vi "SPI_1203v7.vi"() -> ()   [LabVIEW 2018]
uses:
  <vilib>/ni845x/ni845x.llb/ni845xControl.ctl
  <vilib>/ni845x/ni845x.llb/ni845xSpiStreamConfiguration.ctl
  <vilib>/ni845x/ni845x.llb/NI-845x SPI Script Us Delay.vi
  <vilib>/ni845x/ni845x.llb/NI-845x Close Device Reference.vi
  <resource>/objmgr/NI845x.rc
  <vilib>/ptbypt/NI_PtbyPt.lvlib
panel:
  out "СКО":dbl
  out "СЗС":dbl
  in  "Расчет":bool
  in  "ПРИМЕЧАНИЕ":string="1"
  in  "Сохранить кадр":bool
  in  "Frames":path=path "C:/LabView_PRJ/23011_UIC1203R/LabView_PRJ/Frames"
  in  "Waveform1:Timing:T4(drdyA->csA)":u32=20
  in  "RST":bool
  out "Numeric":u32=1
  out "RX BUFFER":string="B0\t58\t75\t52\t00\t00\t00\t00\tB0\t58\t79\t54\t00\t00\t00\t00\tB0\t58\t7D\t55\t00\t00\t00\t00\tB0\t58\t81\t52\t00\t00\t00\t00\tB0\t58\t85\t52\t00\t00\t00\t00\tB0\t58\t89\t50\t00\t00\t00\t00\tB0\t58\t8D\t53\t00\t00\t00\t00\tB0\t58\t91\t4B\t00\t00\t00\t00\tB0\t58\t95\t54\t00\t00\t00\t00\tB0\t58\t99\t4F\t00\t00\t00\t00\tB0\t58\t9D\t4F\t00\t00\t00\t00\tB0\t58\tA1\t4E\t00\t00\t00\t00\tB0\t58\tA5\t4F\t00\t00\t00\t00\tB0\t58\tA9\t50\t00\t00\t00\t00\tB0\t58\tAD\t51\t00\t00\t00\t00\tB0\t58\tB1\t51\t00\t00\t00\t00\tB0\t58\tB5\t4E\t00\t00\t00\t00\tB0\t58\tB9\t4F\t00\t00\t00\t00\tB0\t58\tBD\t4F\t00\t00\t00\t00\tB0\t58\tC1\t4D\t00\t00\t00\t00\tB0\t58\tC5\t4F\t00\t00\t00\t00\tB0\t58\tC9\t50\t00\t00\t00\t00\tB0\t58\tCD\t51\t00\t00\t00\t00\tB0\t58\tD1\t4F\t00\t00\t00\t00\tB0\t58\tD5\t4F\t00\t00\t00\t00\tB0\t58\tD9\t4F\t00\t00\t00\t00\tB0\t58\tDD\t4E\t00\t00\t00\t00\tB0\t58\tE1\t4F\t00\t00\t00\t00\tB0\t58\tE5\t54\t00\t00\t00\t00\tB0\t58\tE9\t4F\t00\t00\t00\t00\tB0\t58\tED\t4F\t00\t00\t00\t00\tB0\t58\tF1\t4D\t00\t00\t00\t00\r\n"
  out "TXBUF":string="90\t00\t00\r\nA0\t02\t82\r\nA1\t0D\t80\r\nA2\t3F\tA3\r\nA3\t3F\t0C\r\nA4\t3E\t80\r\nA5\t3F\tA3\r\nA6\t00\t00\r\nB0\t00\t07\r\nB1\t00\t75\r\nB2\t00\tFF\r\nB3\t00\t0F\r\nB4\t00\t87\r\nB5\t00\tFA\r\nC0\t00\t80\r\nC1\t00\t07\r\n91\t00\t10\r\n92\t00\t02\r\n90\t00\t04\r\n"
  out "S":u16=13389
  out "y":u16=64
  out "x":u16=62
  out "Boolean":bool
  out "Гистограмма яркости по кадру":T1(graph)={"X Values"=array[1023 elements], "Histogram: h(x)"=[1, 11, 0, 9, 0, 63, 0, 109, 0, 199, 332, 0, 461, 0, 478, 0, 472, 0, 517, 446, 0, 396, 0, 337, 0, 279, 0, 300, 228, 0, 238, 0, 216, 0, 245, 0, 198, 191, 0, 177, 0, 158, 0, 120, 0, 138, 144, 0, 122, 0, 89, 0, 84, 0, 99, 0, 73, 59, 0, 38, 0, 25, 0, 29, 0, 20, 21, 0, 17, 0, 20, 0, 12, 0, 5, 9, 0, 2, 0, 7, 0, 4, 0, 6, 4, 0, 10, 0, 4, 0, 5, 0, 4, 5, 0, 3, 0, 4, 0, 1, 0, 4, 0, 4, 1, 0, 4, 0, 5, 0, 6, 0, 3, 3, 0, 1, 0, 0, 0, 1, 0, 3, 1, 0, 4, 0, 3, 0, 1, 0, 2, 2, 0, 2, 0, 1, 0, 3, 0, 3, 1, 0, 1, 0, 4, 0, 0, 0, 2, 0, 0, 2, 0, 0, 0, 1, 0, 2, 0, 0, 3, 0, 5, 0, 1, 0, 1, 0, 0, 2, 0, 0, 0, 0, 0, 3, 0, 1, 0, 0, 2, 0, 0, 0, 0, 0, 2, 1, 0, 2, 0, 1, 0, 0, 0, 0, 0, 0, 2, 0, 1, 0, 0, 0, 1, 0, 2, 1, 0, 1, 0, 1, 0, 2, 0, 0, 0, 0, 0, 0, 0, 0, 1, 0, 2, 2, 0, 1, 0, 1, 0, 2, 0, 0, 0, 0, 0, 0, 0, 0, 0, 0, 1, 0, 1, 1, 0, 0, 0, 0, 0, 0, 0, 0, 0, 0, 1, 0, 3, 0, 1, 0, 1, 0, 0, 0, 0, 0, 0, 1, 0, 0, 0, 0, 0, 0, 0, 0, 2, 0, 2, 1, 0, 1, 0, 1, 0, 0, 0, 0, 1, 0, 2, 0, 2, 0, 0, 0, 0, 0, 2, 0, 0, 3, 0, 0, 0, 1, 0, 2, 1, 0, 0, 0, 1, 0, 2, 0, 0, 2, 0, 1, 0, 0, 0, 0, 0, 0, 1, 0, 1, 0, 1, 0, 1, 0, 1, 1, 0, 0, 0, 1, 0, 1, 0, 1, 0, 0, 0, 0, 0, 0, 0, 0, 1, 0, 0, 0, 0, 0, 0, 0, 0, 2, 0, 1, 0, 0, 1, 0, 1, 0, 0, 0, 0, 0, 0, 0, 0, 0, 0, 1, 0, 2, 1, 0, 0, 0, 0, 0, 0, 0, 1, 0, 1, 0, 0, 2, 0, 0, 0, 0, 0, 2, 1, 0, 1, 0, 0, 0, 1, 0, 1, 2, 0, 1, 0, 1, 0, 0, 0, 0, 2, 0, 1, 0, 0, 0, 1, 0, 0, 2, 0, 0, 0, 2, 0, 0, 0, 1, 0, 0, 0, 0, 1, 0, 0, 0, 0, 0, 0, 1, 0, 0, 0, 1, 0, 2, 0, 3, 1, 0, 0, 0, 1, 0, 1, 0, 0, 0, 0, 2, 0, 1, 0, 0, 0, 1, 1, 0, 2, 0, 0, 0, 0, 0, 0, 0, 2, 1, 0, 3, 0, 0, 0, 0, 0, 1, 2, 0, 3, 0, 0, 0, 0, 0, 0, 0, 0, 0, 0, 0, 0, 2, 0, 0, 0, 0, 0, 0, 0, 0, 1, 0, 1, 1, 0, 0, 0, 2, 0, 0, 0, 0, 2, 0, 0, 0, 1, 0, 0, 0, 0, 0, 0, 2, 0, 0, 0, 0, 0, 0, 0, 0, 0, 0, 0, 0, 0, 0, 1, 0, 1, 0, 0, 1, 0, 1, 0, 0, 0, 0, 0, 0, 1, 0, 0, 0, 1, 0, 0, 0, 0, 1, 0, 1, 0, 0, 0, 0, 0, 0, 0, 0, 0, 0, 0, 0, 1, 0, 0, 0, 0, 0, 0, 1, 0, 2, 0, 0, 0, 0, 0, 0, 1, 0, 0, 0, 1, 1, 0, 1, 0, 0, 0, 0, 0, 0, 0, 0, 1, 0, 1, 0, 1, 0, 0, 0, 1, 0, 0, 0, 0, 0, 0, 0, 0, 1, 0, 0, 0, 0, 2, 0, 2, 0, 2, 0, 0, 1, 0, 1, 0, 0, 0, 1, 2, 0, 0, 0, 0, 0, 1, 0, 0, 0, 0, 0, 0, 1, 0, 0, 0, 0, 0, 0, 1, 0, 1, 0, 1, 0, 0, 0, 2, 0, 0, 1, 0, 0, 0, 0, 0, 0, 1, 0, 2, 0, 3, 0, 1, 0, 0, 0, 0, 1, 0, 0, 0, 1, 0, 0, 1, 0, 1, 0, 1, 0, 1, 0, 0, 0, 0, 1, 0, 0, 0, 0, 0, 1, 0, 0, 1, 0, 0, 0, 0, 0, 0, 0, 0, 0, 0, 1, 0, 0, 0, 0, 0, 2, 0, 0, 1, 0, 1, 0, 0, 0, 0, 0, 0, 0, 0, 0, 0, 0, 0, 1, 0, 0, 0, 0, 0, 0, 0, 0, 0, 0, 1, 0, 0, 1, 0, 0, 0, 0, 0, 1, 1, 0, 0, 0, 1, 0, 0, 0, 0, 0, 0, 1, 0, 0, 0, 1, 0, 0, 0, 0, 0, 0, 0, 0, 0, 0, 0, 0, 0, 0, 0, 0, 0, 0, 0, 0, 0, 0, 0, 0, 0, 0, 0, 0, 0, 0, 0, 0, 0, 0, 0, 0, 0, 0, 0, 0, 0, 0, 0, 0, 0, 0, 0, 0, 0, 0, 0, 0, 0, 0, 0, 0, 0, 0, 0, 0, 0, 0, 0, 0, 0, 0, 0, 0, 0, 0, 0, 0, 0, 0, 0, 0, 0, 0, 0, 0, 0, 0, 0, 0, 0, 0, 0, 0, 0, 0, 0, 0, 0, 0, 0, 0, 0, 0, 0, 0, 0, 0, 0, 0, 0, 0, 0, 0, 0, 1, 0, 0, 0, 0, 0, 0, 0, 0, 0, 0, 0, 0, 0, 0, 0, 0, 0, 0, 0, 1, 0, 0, 0, 0, 0, 0, 0, 0, 0, 0, 0, 0, 0, 1, 0, 0, 0, 0, 0, 0, 0, 0, 0, 0, 0, 0, 0, 0, 0, 0, 0, 0, 0, 0, 0, 0, 0, 0, 0, 0, 0, 0, 0, 0, 0, 0, 0, 0, 0, 0, 0, 0, 0, 0, 0, 0, 0, 0, 0, 0, 0, 0, 0, 0, 0, 0, 0, 0, 0, 0, 0, 0, 0, 0, 0, 0, 0, 0, 1]}
  out "spi stream configuration":T2
  out "device reference out":T3="USB0::0x3923::0x7514::019636F1::RAW"
  out "Run":bool=TRUE
  in  "SaveReg":bool
  in  "Регистры":u8[][](array[numeric])=[[144, 0, 0], [160, 2, 130], [161, 13, 128], [162, 63, 163], [163, 63, 12], [164, 62, 128], [165, 63, 163], [166, 0, 0], [176, 0, 7], [177, 0, 117], [178, 0, 255], [179, 0, 15], [180, 0, 135], [181, 0, 250], [192, 0, 128], [193, 0, 7], [145, 0, 16], [146, 0, 2], [144, 0, 4]] format="%02x"
  in  "stop":bool=TRUE
  out "Строка":u32=44 format="%x"
  out "Столбец":u32=60 format="%x"
  out "Фоновый кадр":u16[][](graph)
  out "24бита":u32=5828941 format="%x"
  out "Яркость":u32=333
  out "Адрес":u32=5692 format="%x"
  out "Состояние":T4={"SEU"=FALSE, "OVR"=TRUE, "RDY"=TRUE, "N"=0}
  # "CONTROL[2]\nTC_RST\nTC_F1\nTC_TX\nTC_F2\nTC_CS\nTC_EKL\nRTM[0]\nKODR[3:0]\nKODW[7:0]\nKODT[7:0]\nRUNB[3:0]\nDRES[7:0]\nKODV[0:7]\nPOR[9:0]\nRAF[2:0]\nCONFIG[15:4]\nEXP[15:0]\nCONTROL[2]"
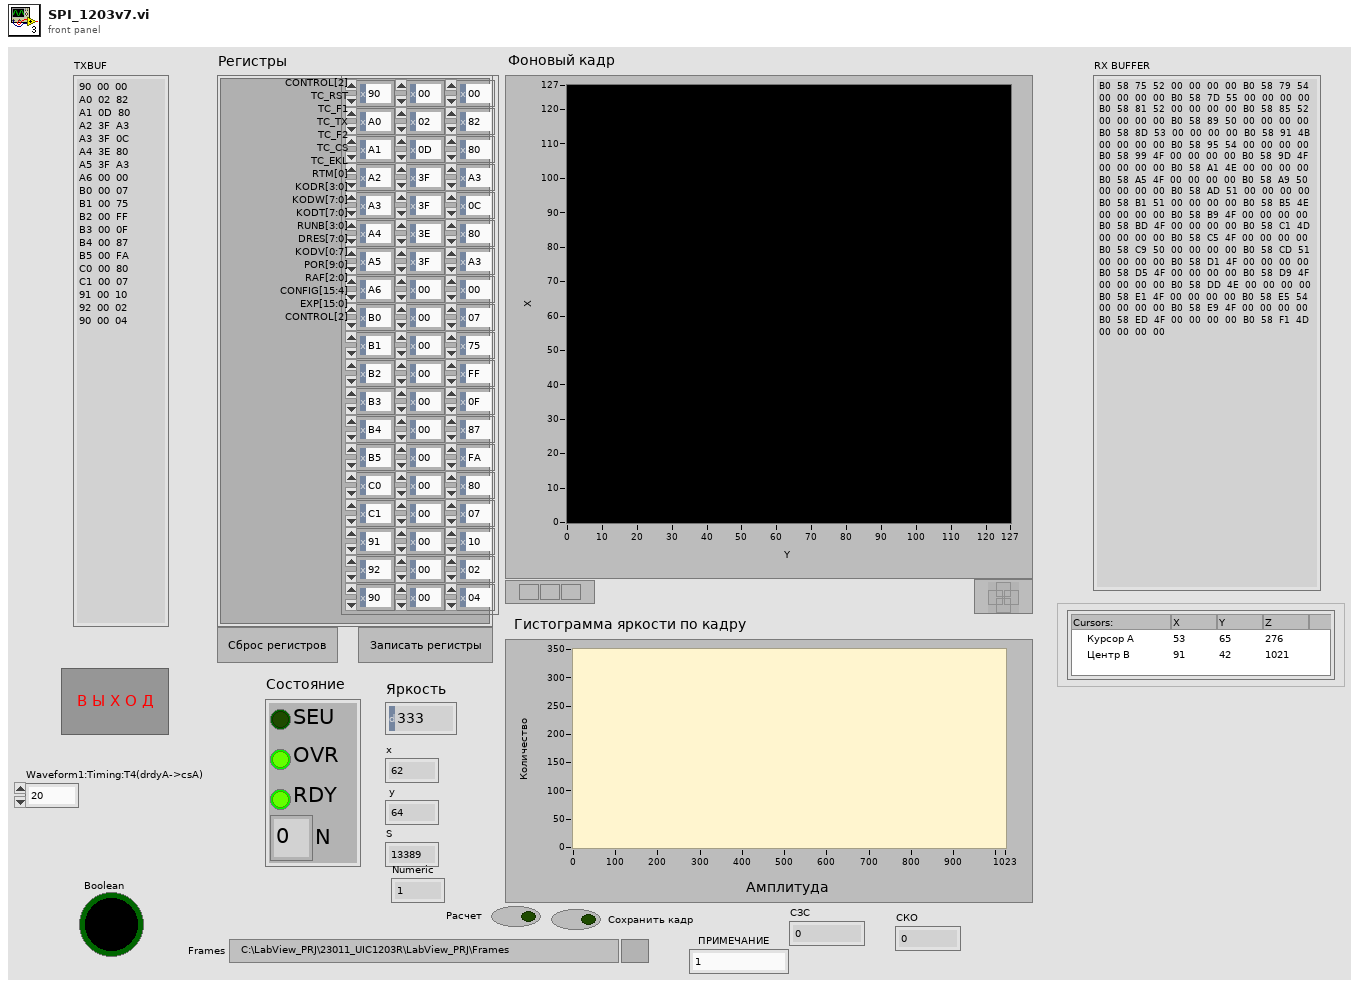
[diagram p1: front panel]
types:
  T1 = cluster{"X Values":dbl[], "Histogram: h(x)":i32[]}
  T2 = typedef "ni845xSpiStreamConfiguration.ctl" = refnum<k20>
  T3 = typedef "ni845xControl.ctl" = refnum<k21>
  T4 = cluster{"SEU":bool, "OVR":bool, "RDY":bool, "N":u8}
  T5 = typedef "Image Type" = u32
  T6 = typedef "IMAQ Image.ctl" = refnum<image>
  T7 = typedef "ni845xSpiScriptControl.ctl" = refnum<k20>
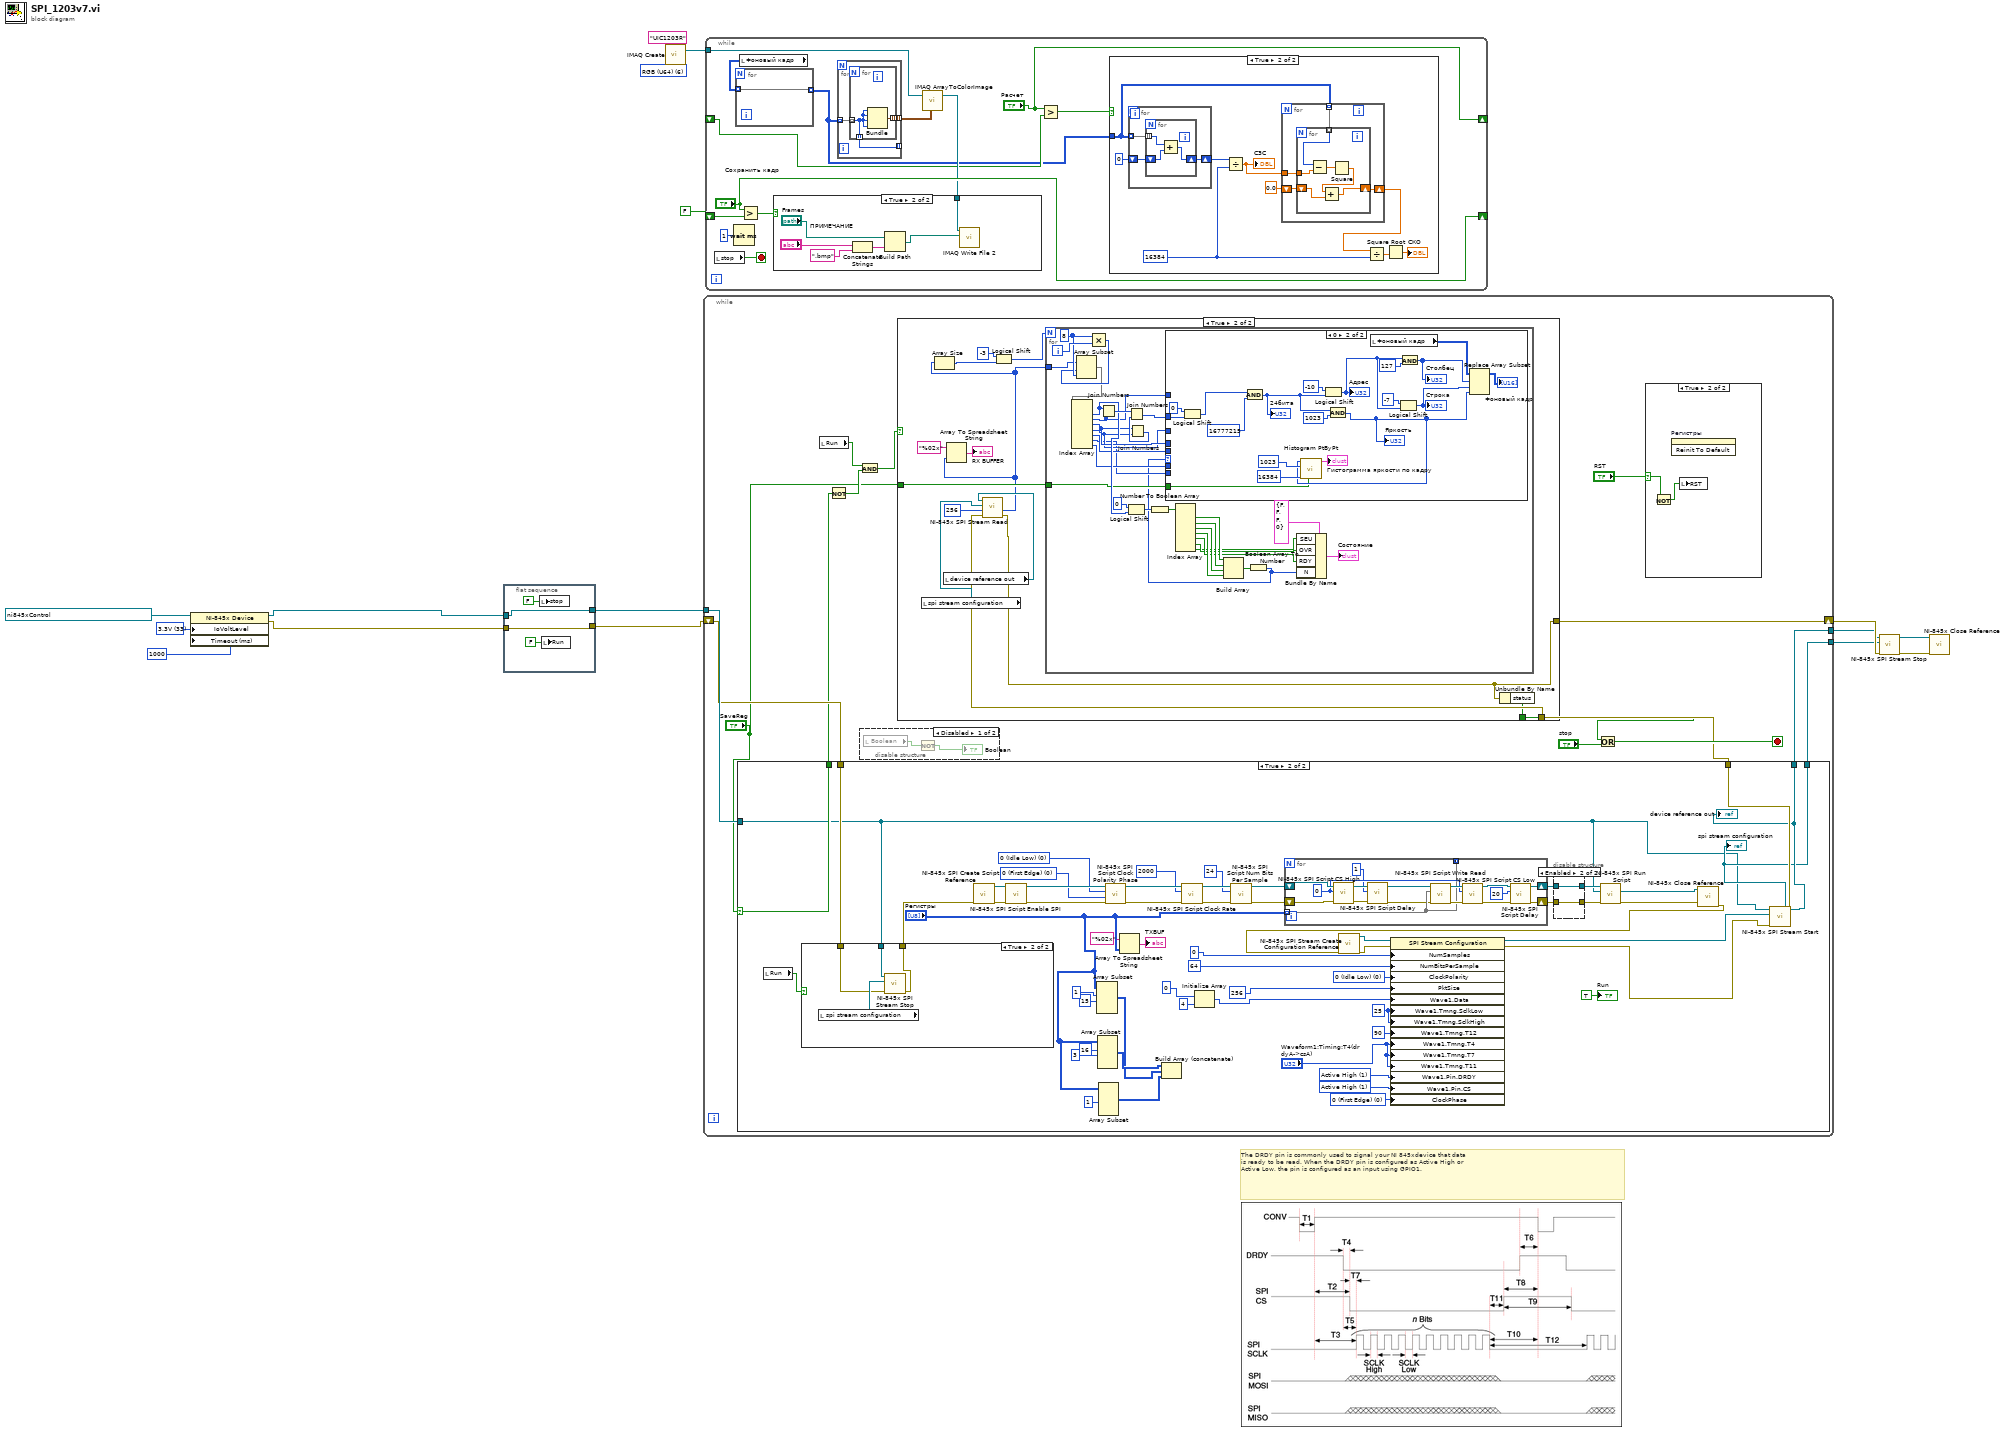
[diagram p0: block diagram]
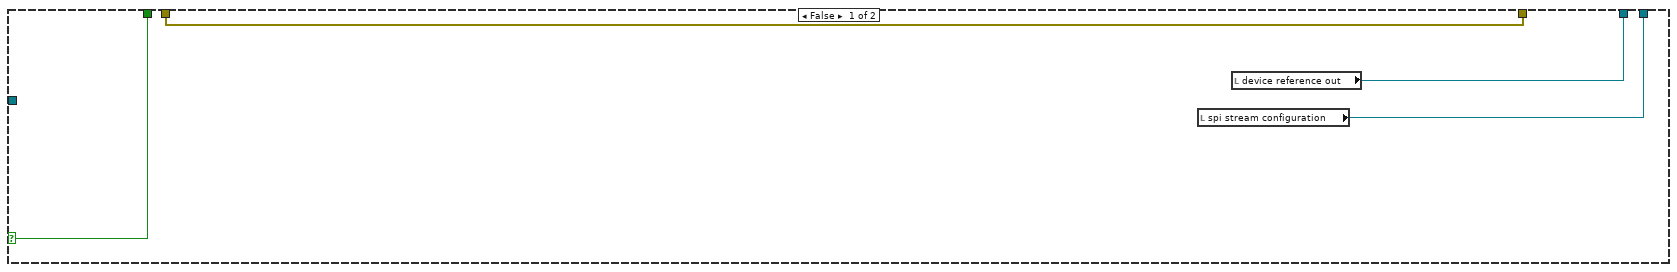
[diagram p6: hidden frame]
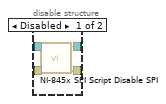
[diagram p7: hidden frame]
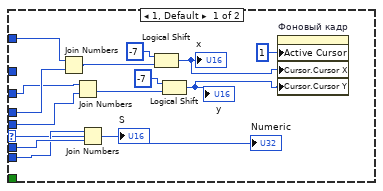
[diagram p10: hidden frame]
diagram:
  w3 = T5 6 items=["Grayscale (U8)", "Grayscale (I16)", "Grayscale (SGL)", "Complex (CSG)", "RGB (U32)", "HSL (U32)", "RGB (U64)"] ("Image Type")
  w16 = 33 items=["3.3V"=33, "2.5V"=25, "1.8V"=18, "1.5V"=15, "1.2V"=12] ("I/O Voltage Level")
  # "The DRDY pin is commonly used to signal your NI 845xdevice that data \nis ready to be read. When the DRDY pin is configured as Active High or \nActive Low, the pin is configured as an input using GPIO1."
  n1 = property class="NI-845x Device"(reference=T3 "USB0::0x3923::0x7514::019636F1::RAW" ("device reference"), "IoVoltLevel"=w16, "Timeout (ms)"=u32 1000 ("Timeout Value (ms)")) -> (reference out=w11:T3, error out=w9:errorcluster)  [unwired: 1 in]
  n2 = flat-sequence {
    tunnel: [w20] -> w10
    tunnel: w11 -> [w20]
    tunnel: [w18] -> w8
    tunnel: w9 -> [w18]
    frame #0 {
      n3 = local write "stop"(FALSE ("stop")) -> ()
      n4 = local write "Run"(FALSE ("Run")) -> ()
    }
  }
  n5 = call "IMAQ Create"("Image Name"="UIC1203R", "Image Type"=w3) -> ("New Image"=w1:T6)  [unwired: 3 in, 1 out]
  n6 = while {
    tunnel: w10 -> [w33]
    shift-right: [w30] -> w12
    shift-left: w8 -> [w32]
    tunnel: [w28] -> w6
    tunnel: [w27] -> w7
    stop <- w34 stop-if-true
    n7 = case shown="True" "SaveReg" {
      selector: "SaveReg" -> [w40 w70]
      tunnel: w33 -> [_ w63]
      tunnel: w32 -> [w43 w68]
      tunnel: [w43 w73] -> w31
      tunnel: [w42 w72] -> w28
      tunnel: [w41 w71] -> w27
      tunnel: [w40 w70] -> w23
      frame False {
        n8 = local read "spi stream configuration"() -> (w41:T2)
        n9 = local read "device reference out"() -> (w42:T3)
      }
      frame True {
        w61 = 0 items=["0 (First Edge)", "1 (Second Edge)"] ("clock phase (0)")
        w62 = 0 items=["0 (Idle Low)", "1 (Idle High)"] ("clock polarity (0)")
        w65 = u8 1 items=["Disabled", "Active High", "Active Low"] ("Waveform1:Pin:DRDY")
        w66 = u8 0 items=["0 (First Edge)", "1 (Second Edge)"] ("Clock Phase")
        w80 = u8 1 items=["Disabled", "Active High", "Active Low"] ("Waveform1:Pin:DRDY")
        w81 = u32 25 ("Waveform1:Timing:SCLKLow")
        w85 = u8 0 items=["0 (Idle Low)", "1 (Idle High)"] ("Clock Polarity")
        n10 = local read "Run"() -> (w69:bool)
        n11 = case shown="True" w69 {
          tunnel: w63 -> [_ w112]
          tunnel: w68 -> [w108 w110]
          tunnel: [w108 w109] -> w67
          frame False {
          }
          frame True {
            n12 = local read "spi stream configuration"() -> (w111:T2)
            n13 = call <vilib>:"NI-845x SPI Stream Stop.vi"("error in (no error)"=w110, "spi stream configuration in"=w111, "device reference in"=w112) -> ("error out"=w109:errorcluster)  [unwired: 6 in, 2 out]
          }
        }
        n14 = call <vilib>:"NI-845x SPI Create Script Reference.vi"("error in (no error)"=w67) -> ("error out"=w101:errorcluster, "spi script reference"=w64:T7)  [unwired: 9 in]
        n15 = call <vilib>:"NI-845x SPI Script Enable SPI.vi"("error in (no error)"=w101, "spi script reference in"=w64) -> ("error out"=w100:errorcluster, "spi script reference out"=w99:T7)  [unwired: 8 in]
        n16 = Array Subset(array="Регистры", index (row)=1, length (row)=15 ("length")) -> (w48:u8[][])  [unwired: 2 in]
        n17 = Array Subset(array="Регистры", index (row)=16 ("index"), length (row)=3 ("length")) -> (w49:u8[][])  [unwired: 2 in]
        n18 = Array Subset(array="Регистры", length (row)=1 ("length")) -> (w47:u8[][])  [unwired: 3 in]
        n19 = call <vilib>:"NI-845x SPI Script Clock Polarity Phase.vi"("error in (no error)"=w100, "clock phase (0)"=w61, "clock polarity (0)"=w62, "spi script reference in"=w99) -> ("error out"=w98:errorcluster, "spi script reference out"=w97:T7)  [unwired: 6 in]
        n20 = Array To Spreadsheet String(array="Регистры", 3:"%02x" ("format string")) -> (spreadsheet string=→"TXBUF":string)  [unwired: 1 in]
        n21 = Build Array (concatenate)(w49, w48, w47) -> ()  [unwired: 1 out]
        n22 = call <vilib>:"NI-845x SPI Script Clock Rate.vi"("error in (no error)"=w98, "clock rate in kHz (1000)"=u16 2000, "spi script reference in"=w97) -> ("error out"=w94:errorcluster, "spi script reference out"=w95:T7)  [unwired: 7 in]
        n23 = Initialize Array(u8 0 ("chip select (0)"), 4 ("dimension size")) -> (w83:u8[])
        n24 = call <vilib>:"NI-845x SPI Script Num Bits Per Sample.vi"("error in (no error)"=w94, "num bits per sample (8)"=u16 24, "spi script reference in"=w95) -> ("error out"=w55:errorcluster, "spi script reference out"=w56:T7)  [unwired: 7 in]
        n25 = for {
          shift-right: [w119] -> w90
          shift-left: w55 -> [w128]
          shift-right: [w120] -> w91
          shift-left: w56 -> [w127]
          tunnel: "Регистры" -> [w118] mode=indexing
          tunnel: [w118] -> _ mode=concatenating
          w124 = u32 0 ("chip select (0)")
          n26 = call <vilib>:"NI-845x SPI Script CS High.vi"("error in (no error)"=w128, "chip select (0)"=w124, "spi script reference in"=w127) -> ("error out"=w117:errorcluster, "spi script reference out"=w116:T7)  [unwired: 7 in]
          n27 = call-poly <vilib>:"NI-845x SPI Script Delay.vi"("error in (no error)"=w117, "delay in microseconds (0)"=u16 1, "spi script reference in"=w116) -> ("error out"=w114:errorcluster, "spi script reference out"=w115:T7)  [unwired: 7 in]
          n28 = call <vilib>:"NI-845x SPI Script Write Read.vi"("error in (no error)"=w114, "write data"=w118, "spi script reference in"=w115) -> ("error out"=w126:errorcluster, "spi script reference out"=w125:T7)  [unwired: 6 in, 1 out]
          n29 = call <vilib>:"NI-845x SPI Script CS Low.vi"("error in (no error)"=w126, "chip select (0)"=w124, "spi script reference in"=w125) -> ("error out"=w122:errorcluster, "spi script reference out"=w123:T7)  [unwired: 7 in]
          n30 = call-poly <vilib>:"NI-845x SPI Script Delay.vi"("error in (no error)"=w122, "delay in microseconds (0)"=u8 20 ("delay in milliseconds (0)"), "spi script reference in"=w123) -> ("error out"=w119:errorcluster, "spi script reference out"=w120:T7)  [unwired: 7 in]
        }
        n31 = disable-structure shown="Enabled" {
          disable-tunnel: [w105 w106] -> w93
          disable-tunnel: [w104 w107] -> w92
          disable-tunnel: w91 -> [w103 w107]
          disable-tunnel: w90 -> [w102 w106]
          frame Disabled {
            n32 = call <vilib>:"NI-845x SPI Script Disable SPI.vi"("error in (no error)"=w102, "spi script reference in"=w103) -> ("error out"=w105:errorcluster, "spi script reference out"=w104:T7)  [unwired: 8 in]
          }
          frame Enabled {
          }
        }
        n33 = call <vilib>:"NI-845x SPI Run Script.vi"("error in (no error)"=w93, "device reference in"=w63, "spi script reference in"=w92) -> ("error out"=w89:errorcluster, "device reference out"=w60:T3)  [unwired: 6 in, 1 out]
        n34 = call-poly <vilib>:"NI-845x Close Reference.vi"("error in (no error)"=w89, "device reference"=w60) -> ("error out"=w77:errorcluster)  [unwired: 9 in]
        n35 = call <vilib>:"NI-845x SPI Stream Create Configuration Reference.vi"("error in (no error)"=w77) -> ("error out"=w82:errorcluster, "spi stream configuration"=w87:T2)  [unwired: 9 in]
        n36 = property class="SPI Stream Configuration"(reference=w87, error in=w82, "NumSamples"=u32 0 ("Number of Samples"), "NumBitsPerSample"=u8 64 ("Number of Bits Per Sample"), "ClockPolarity"=w85, "PktSize"=u32 256 ("Packet Size"), "Wave1.Data"=w83, "Wave1.Tmng.SclkLow"=w81, "Wave1.Tmng.SclkHigh"=w81, "Wave1.Tmng.T12"=u32 90 ("Waveform1:Timing:T12(sclkD->sclkA)"), "Wave1.Tmng.T4"="Waveform1:Timing:T4(drdyA->csA)", "Wave1.Tmng.T7"="Waveform1:Timing:T4(drdyA->csA)", "Wave1.Tmng.T11"="Waveform1:Timing:T4(drdyA->csA)", "Wave1.Pin.DRDY"=w80, "Wave1.Pin.CS"=w65, "ClockPhase"=w66) -> (reference out=w74:T2, error out=w76:errorcluster)
        n37 = call <vilib>:"NI-845x SPI Stream Start.vi"("error in (no error)"=w76, "spi stream configuration in"=w74, "device reference in"=w63) -> ("error out"=w73:errorcluster, "spi stream configuration out"=w71:T2, "device reference out"=w72:T3)  [unwired: 6 in]
        "device reference out" <- w72
        "spi stream configuration" <- w71
        "Run" <- TRUE ("Run")
      }
    }
    n38 = local read "Run"() -> (w25:bool)
    n39 = Not(x=w23) -> (.not. x?=w26:bool)
    n40 = disable-structure shown="Disabled" {
      frame Disabled {
        n41 = local read "Boolean"() -> (w39:bool)
        n42 = Not(x=w39) -> (.not. x?=→"Boolean":bool)
      }
      frame Enabled {
      }
    }
    n43 = And(x=w25, y=w26) -> (x .and. y?=w24:bool)
    n44 = case shown="True" w24 {
      tunnel: w31 -> [w129 w138]
      tunnel: [w129 w137] -> w30
      tunnel: [_ w136] -> w29
      tunnel: "SaveReg" -> [_ w134]
      frame False {
      }
      frame True {
        n45 = local read "spi stream configuration"() -> (w139:T2)
        n46 = local read "device reference out"() -> (w140:T3)
        n47 = call <vilib>:"NI-845x SPI Stream Read.vi"("error in (no error)"=w138, "num bytes per read"=256, "spi stream configuration in"=w139, "device reference in"=w140) -> ("error out"=w137:errorcluster, "read data"=w130:u8[])  [unwired: 4 in, 2 out]
        n48 = Array Size(array=w130) -> (size(s)=w142:i32)
        n49 = Array To Spreadsheet String(array=w130, 3:"%02x" ("format string")) -> (spreadsheet string=→"RX BUFFER":string)  [unwired: 1 in]
        n50 = Logical Shift(y=i16 -3, x=w142) -> (x << y=w135:i32)
        n51 = for {
          N: w135 -> [_]
          tunnel: w130 -> [w153]
          tunnel: w134 -> [w151]
          i -> [w169]
          w168 = 8 ("length")
          n52 = Multiply(x=w168, y=w169) -> (x*y=w167:i32)
          n53 = Array Subset(array=w153, index=w167, length=w168) -> (w144:u8[])
          n54 = Index Array(array=w144) -> (element #1=w152:u8, element #2=w150:u8, element #3=w149:u8, element #4=w148:u8, element #5=w147:u8, element #6=w145:u8, element #7=w146:u8)  [unwired: 7 in]
          n55 = Join Numbers(hi=w152, lo=w150) -> ((hi.lo)=w172:u16)
          n56 = Logical Shift(y=i16 0, x=w152) -> (x << y=w154:u8)
          n57 = Join Numbers(hi=w149, lo=w148) -> ((hi.lo)=w171:u16)
          n58 = Join Numbers(hi=w172, lo=w171) -> ((hi.lo)=w170:u32)
          n59 = Number To Boolean Array(number=w154) -> (Boolean array=w166:bool[])
          n60 = Index Array(array=w166) -> (element #1=w163:bool, element #2=w162:bool, element #3=w161:bool, element #4=w160:bool, element #5=w159:bool, element #6=w158:bool, element #7=w157:bool)  [unwired: 7 in]
          n61 = Build Array(w163, w162, w161, w160) -> (w156:bool[])
          n62 = Boolean Array To Number(Boolean array=w156) -> (number=w143:u32)
          n63 = case shown="0" w143 {
            selector: w143 -> [w176 _]
            tunnel: w170 -> [_ w204]
            tunnel: w151 -> [_ w188]
            tunnel: w150 -> [w182 _]
            tunnel: w149 -> [w183 _]
            tunnel: w148 -> [w180 _]
            tunnel: w147 -> [w181 _]
            tunnel: w146 -> [w179 _]
            tunnel: w145 -> [w178 _]
            frame 1, Default {
              n64 = Join Numbers(hi=w182, lo=w183) -> ((hi.lo)=w186:u16)
              n65 = Join Numbers(hi=w180, lo=w181) -> ((hi.lo)=w184:u16)
              n66 = Join Numbers(hi=w178, lo=w179) -> ((hi.lo)=→"S":u16)
              n67 = Logical Shift(y=i16 -7, x=w186) -> (x << y=w174:u16)
              "x" <- w174
              n68 = Logical Shift(y=i16 -7, x=w184) -> (x << y=w173:u16)
              "y" <- w173
              n69 = property on="Фоновый кадр" class="IntGraph (strict)"("Active Cursor"=u32 1, "Cursor.Cursor X"=w174, "Cursor.Cursor Y"=w173) -> ()  [unwired: 2 in, 2 out]
              "Numeric" <- w176
            }
            frame 0 {
              n70 = Logical Shift(y=i16 0, x=w204) -> (x << y=w202:u32)
              n71 = And(x=w202, y=u32 16777215) -> (x .and. y?=w200:u32)
              "24бита" <- w200
              n72 = Logical Shift(y=i16 -10, x=w200) -> (x << y=w195:u32)
              "Адрес" <- w195
              n73 = And(x=w200, y=u32 1023) -> (x .and. y?=w189:u32)
              "Яркость" <- w189
              n74 = call <vilib>:"Histogram PtByPt.vi"("initialize"=w188, "sample length"=16384, "intervals"=1023, "x"=w189) -> ("Histogram Graph"=→"Гистограмма яркости по кадру":T1)  [unwired: 4 in, 3 out]
              n75 = local read "Фоновый кадр"() -> (w196:u16[][])
              n76 = Logical Shift(y=i16 -7, x=w195) -> (x << y=w194:u32)
              "Строка" <- w194
              n77 = And(x=w195, y=u32 127) -> (x .and. y?=w193:u32)
              "Столбец" <- w193
              n78 = Replace Array Subset(array=w196, new element=w189, index (row)=w193, index (col)=w194) -> (→"Фоновый кадр":u16[][])
            }
          }
          n79 = Bundle By Name(cluster=T4 {"SEU"=FALSE, "OVR"=FALSE, "RDY"=FALSE, "N"=0} ("Cluster"), "SEU"=w157, "OVR"=w158, "RDY"=w159, "N"=w143) -> (→"Состояние":T4)
        }
        n80 = Unbundle By Name(w137) -> ("status"=w136:bool)
      }
    }
    n81 = Or(x=w29, y="stop") -> (x .or. y?=w34:bool)
    n82 = case shown="True" "RST" {
      selector: "RST" -> [_ w37]
      frame False {
      }
      frame True {
        n83 = Not(x=w37) -> (.not. x?=w36:bool)
        n84 = invoke on="Регистры" class="Arr (strict)" method="Reinit To Default"() -> ()  [unwired: 3 in, 3 out]
        n85 = local write "RST"(w36) -> ()
      }
    }
  }
  n86 = while {
    shift-right: ["Сохранить кадр"] -> _
    shift-left: FALSE -> [w217]
    tunnel: w1 -> [w212]
    shift-right: ["Расчет"] -> _
    shift-left: _ -> [w209]
    stop <- w219 stop-if-true
    n87 = local read "stop"() -> (w219:bool)
    n88 = Wait (ms)(milliseconds to wait=u32 1) -> ()  [unwired: 1 out]
    n89 = local read "Фоновый кадр"() -> (w214:u16[][])
    n90 = for {
      tunnel: w214 -> [w250] mode=indexing
      tunnel: [w250] -> w207 mode=indexing
    }
    n91 = Greater?(x="Сохранить кадр", y=w217) -> (0:w215:bool)
    n92 = for {
      tunnel: [w247] -> w213 mode=indexing
      tunnel: w207 -> [w246] mode=indexing
      tunnel: [w245] -> _ mode=indexing
      n93 = for {
        tunnel: w246 -> [w248] mode=indexing
        tunnel: [w249] -> w247 mode=indexing
        tunnel: [w248] -> w245 mode=indexing
        n94 = Bundle(w248, w248, w248, w248) -> (w249:cluster{u16, u16, u16, u16})  [unwired: 1 in]
      }
    }
    n95 = call "IMAQ ArrayToColorImage"("Image"=w212, "Image Pixels (U64)"=w213) -> ("Image Out"=w211:T6)  [unwired: 3 in, 1 out]
    n96 = case shown="True" w215 {
      tunnel: w211 -> [_ w251]
      frame False {
      }
      frame True {
        n97 = Concatenate Strings("ПРИМЕЧАНИЕ", ".bmp" ("name or relative path")) -> (w253:string)
        n98 = Build Path(base path="Frames", name or relative path=w253) -> (appended path=w252:path)
        n99 = call-poly "IMAQ Write File 2"("File Path"=w252, "Image"=w251) -> ()  [unwired: 8 in, 2 out]
      }
    }
    n100 = Greater?(x="Расчет", y=w209) -> (0:w208:bool)
    n101 = case shown="True" w208 {
      tunnel: w207 -> [_ w224]
      frame False {
      }
      frame True {
        w220 = 16384
        n102 = for {
          tunnel: w224 -> [w239] mode=indexing
          shift-right: [w240] -> w227
          shift-left: 0 -> [w241]
          n103 = for {
            tunnel: w239 -> [w244] mode=indexing
            shift-right: [w242] -> w240
            shift-left: w241 -> [w243]
            n104 = Add(x=w244, y=w243) -> (x+y=w242:i32)
          }
        }
        n105 = Divide(x=w227, y=w220) -> (x/y=w223:dbl)
        "СЗС" <- w223
        n106 = for {
          tunnel: w224 -> [w232] mode=indexing
          tunnel: w223 -> [w231]
          shift-right: [w229] -> w221
          shift-left: 0.0 -> [w230]
          n107 = for {
            tunnel: w232 -> [w238] mode=indexing
            tunnel: w231 -> [w237]
            shift-right: [w233] -> w229
            shift-left: w230 -> [w234]
            n108 = Subtract(x=w238, y=w237) -> (x-y=w236:dbl)
            n109 = Square(x=w236) -> (x^2=w235:dbl)
            n110 = Add(x=w235, y=w234) -> (x+y=w233:dbl)
          }
        }
        n111 = Divide(x=w221, y=w220) -> (x/y=w225:dbl)
        n112 = Square Root(x=w225) -> (sqrt(x)=→"СКО":dbl)
      }
    }
  }
  n113 = call <vilib>:"NI-845x SPI Stream Stop.vi"("error in (no error)"=w12, "spi stream configuration in"=w7, "device reference in"=w6) -> ("error out"=w14:errorcluster, "device reference out"=w13:T3)  [unwired: 6 in, 1 out]
  n114 = call-poly <vilib>:"NI-845x Close Reference.vi"("error in (no error)"=w14, "device reference"=w13) -> ()  [unwired: 9 in, 1 out]
